vi "Enable Custom Device.vi"(8 "error in":errorcluster, 11 "custom device ref in":T1 format="%.0x") -> (0 "error out":errorcluster, 3 "custom device ref out":T1 format="%.0x")   [LabVIEW 2020, in "AIM ARINC 664 Scripting.lvlib"]
doc: "Enables an AIM ARINC 664 custom device."
uses:
  AIM ARINC 664 Scripting.lvlib
  Constants.vi
  <vilib>/NI VeriStand/Custom Device API/Custom Device API.lvlib
  NationalInstruments.VeriStand.SystemDefinitionAPI
  <vilib>/NI VeriStand/Custom Device API/Custom Device Item Ref.ctl
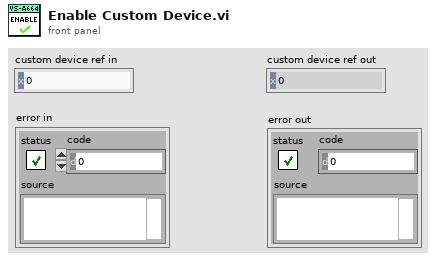
[diagram p1: front panel]
types:
  T1 = typedef "Custom Device API.lvlib/Custom Device Item Ref.ctl" = u64
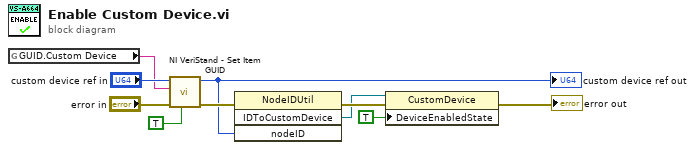
[diagram p0: block diagram]
diagram:
  n1 = global read "Constants.vi" "GUID.Custom Device"() -> (w9:string)
  n2 = call <vilib>:"NI VeriStand - Set Item GUID.vi"("Refresh System Explorer Tree? (F)"=TRUE, "error in (no error)"="error in", "GUID"=w9, "Item Ref in"="custom device ref in") -> ("error out"=w6:errorcluster, "Item Ref out"=w5:T1)  [unwired: 6 in]
  "custom device ref out" <- w5
  n3 = invoke class="NodeIDUtil" method="IDToCustomDevice"(error in=w6, "nodeID"=w5) -> (error out=w4:errorcluster, "IDToCustomDevice"=w3:refnum<k24>)  [unwired: 2 in, 2 out]
  n4 = property class="CustomDevice"(reference=w3, error in=w4, "DeviceEnabledState"=TRUE) -> (error out=→"error out":errorcluster)  [unwired: 1 out]
